vi "split_tdms.vi"() -> ()   [LabVIEW 2018]
panel:
  out "文件结束？":bool
  in  "一次读取的最大数目":i64=6000000
  in  "file path of Smaller TDMS Files":path=path "D:/数据转换/FTIR_"
  in  "file path of Large TDMS File":path=path "D:/数据转换/FTIR.tdms"
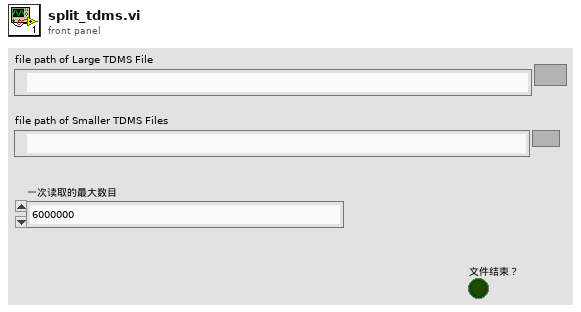
[diagram p1: front panel]
types:
  T1 = enum16{"open", "open or create", "create or replace", "create", "open (read-only)"}
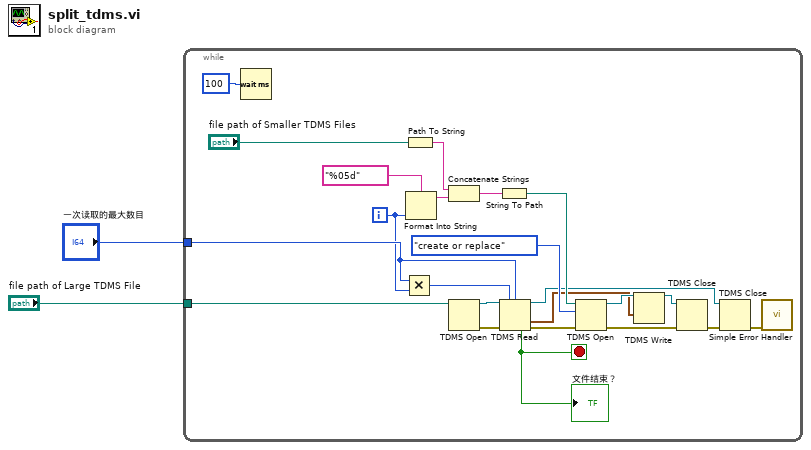
[diagram p0: block diagram]
diagram:
  n1 = while {
    tunnel: "一次读取的最大数目" -> [w13]
    tunnel: "file path of Large TDMS File" -> [w9]
    i -> [w5]
    stop <- w6 stop-if-true
    n2 = Wait (ms)(milliseconds to wait=u32 100) -> ()  [unwired: 1 out]
    n3 = Multiply(x=w13, y=w5) -> (x*y=w12:i64)
    n4 = Path To String(path="file path of Smaller TDMS Files") -> (string=w24:string)
    n5 = Format Into String(format string="%05d" ("格式字符串"), w5) -> (resulting string=w3:string)  [unwired: 2 in, 1 out]
    n6 = Concatenate Strings(w24, w3) -> (w23:string)
    n7 = TDMS Open(11:w9) -> (0:w14:errorcluster, 3:w16:refnum<k34>)  [unwired: 6 in]
    n8 = String To Path(string=w23) -> (path=w22:path)
    n9 = TDMS Read(0:w16, 1:w12, 2:w13, 11:w14) -> (4:w15:refnum<k34>, 10:w8:waveform(dbl)[], 14:w6:bool, 15:w7:errorcluster)  [unwired: 4 in, 2 out]
    "文件结束？" <- w6
    n10 = TDMS Open(8:w7, 10:T1."create or replace" ("operation (0:open)"), 11:w22) -> (0:w20:errorcluster, 3:w11:refnum<k34>)  [unwired: 4 in]
    n11 = TDMS Write(0:w11, 9:w8) -> (4:w10:refnum<k34>)  [unwired: 4 in, 3 out]
    n12 = TDMS Close(8:w20, 11:w10) -> (0:w19:errorcluster)  [unwired: 1 out]
    n13 = TDMS Close(8:w19, 11:w15) -> (0:w18:errorcluster)  [unwired: 1 out]
    n14 = call <vilib>:"Simple Error Handler.vi"("error in (no error)"=w18) -> ()  [unwired: 4 in, 5 out]
  }
